vi "Log Counts.vi"(8 "error in (no error)":errorcluster, 9 "Message":string, 10 "Counts":dbl, 11 "Particle Counter in":refnum<class "Particle Counter.lvclass">) -> (0 "error out":errorcluster, 3 "Particle Counter out":refnum<class "Particle Counter.lvclass">)   [LabVIEW 2023, in "Particle Counter.lvlib" / "Particle Counter.lvclass"]
uses:
  Particle Counter.lvclass
  Particle Counter.lvclass/Particle Counter.ctl
  Application Messages/Viewer Status Message Msg/Viewer Status Message Msg.lvclass
  <vilib>/ActorFramework/Actor/Actor.lvclass
  C:/Program Files/National Instruments/LabVIEW 2023/vi.lib/ActorFramework/Actor/Actor.lvclass
  C:/FlashGordon/Development/Services/Particle Counter/Particle Counter/Particle Counter.lvclass
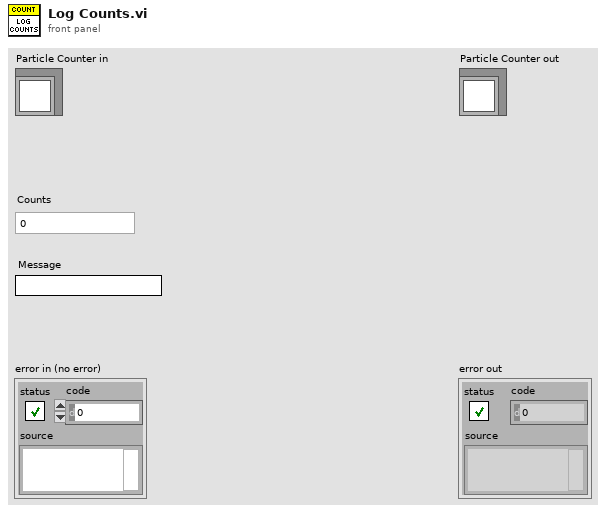
[diagram p1: front panel]
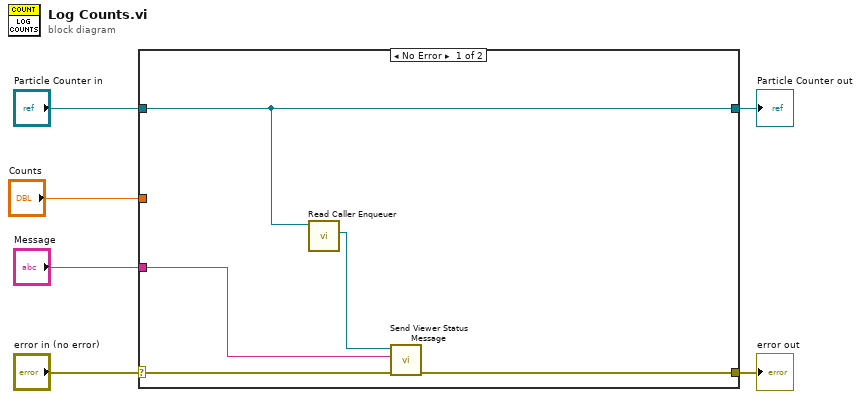
[diagram p0: block diagram]
diagram:
  n1 = case shown="No Error" "error in (no error)" {
    selector: "error in (no error)" -> [w11 w13]
    tunnel: [w7 w13] -> w5
    tunnel: [w8 w12] -> w3
    tunnel: "Particle Counter in" -> [w8 w12]
    tunnel: "Counts" -> [_ _]
    tunnel: "Message" -> [w10 _]
    frame No Error {
      n2 = call <vilib>:"Read Caller Enqueuer.vi"("Actor"=w8) -> ("Caller Enqueuer"=w9:refnum<class "Message Enqueuer.lvclass">)  [unwired: 10 in]
      n3 = call "Send Viewer Status Message.vi"("error in (no error)"=w11, "Message"=w10, "Message Enqueuer"=w9) -> ("error out"=w7:errorcluster)  [unwired: 7 in, 1 out]
    }
    frame Error {
    }
  }
  "error out" <- w5
  "Particle Counter out" <- w3
